vi "Tracking_End.vi"(6 "Last Frame Data":T3 {"Frame Data"."Image Type" items=["Grayscale (U8)", "Grayscale (I16)", "Grayscale (SGL)", "Complex (CSG)", "RGB (U32)", "HSL (U32)", "RGB (U64)", "Grayscale (U16)"]}, 7 "?":T1, 8 "error in":errorcluster, 9 "Settings":T5={"Harware Configuration"={"Camera"="cam1", "Frames Per Second"=15, "Simulate Recording"=FALSE, "Simulated Recording Sample"=path "", "Timestamp Method"=enum."Camera Timestamp"}, "Base Recording Path"=path "", "Type Of Recording"="", "Recording Codec"="", "TrackingSettings"={"Max Radius"=0, "Threshold"=255.0, "ROI"={"Left"=1, "Top"=1, "Right"=2, "Bottom"=0, "Rotation"=0.0}}, "Calibration"={"Pixel Width (X)"=1.0, "Pixel Height (Y)"=1.0}, "Broadcast Length"=0} {"Broadcast Length" min=0; "TrackingSettings"."ROI"."Rotation" format="%.2f"; "TrackingSettings"."ROI"."Left" scale=0.0..1024.0; "TrackingSettings"."ROI"."Right" scale=0.0..1024.0; "TrackingSettings"."Threshold" scale=0.0..255.0}, 10 "Output Data Queue":refnum<queue>, 11 "Input Data Queue":refnum<queue>) -> (0 "error out":errorcluster, 2 "Output Data Queue":refnum<queue>, 3 "Input Data Queue 2":refnum<queue>, 4 "Last Frame Data Out":T3 {"Frame Data"."Image Type" items=["Grayscale (U8)", "Grayscale (I16)", "Grayscale (SGL)", "Complex (CSG)", "RGB (U32)", "HSL (U32)", "RGB (U64)", "Grayscale (U16)"]}, 5 "?":T1)   [LabVIEW 2017, in "ImageAcquisitionLibrary.lvlib"]
uses:
  ImageAcquisitionLibrary.lvlib
  Acquisition/AcquireData.ctl
  Settings/Settings.ctl
  <vilib>/userdefined/High Color/IMAQdx.ctl
  TrackingSettings.ctl
  Settings/Calibration.ctl
  TrackingImages.ctl
  <vilib>/vision/Image Controls.llb/IMAQ Image.ctl
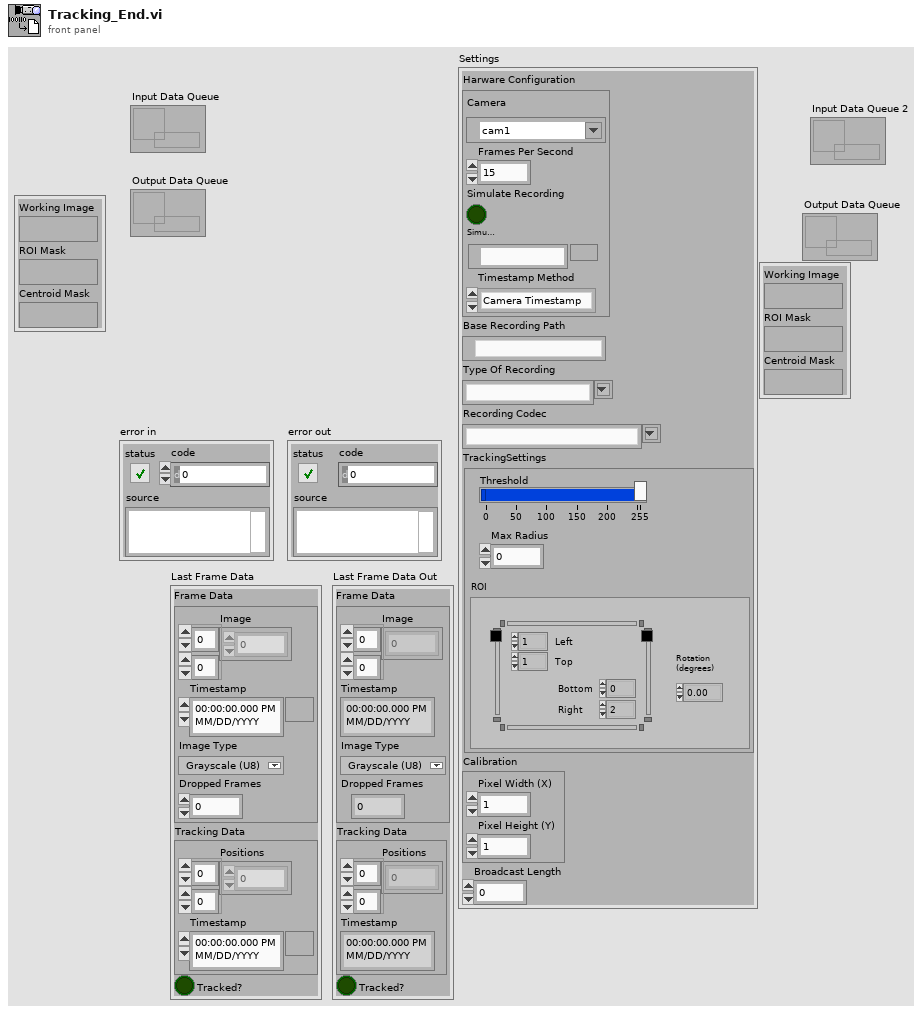
[diagram p1: front panel]
types:
  T1 = typedef "ImageAcquisitionLibrary.lvlib/TrackingImages.ctl" = cluster{"Working Image":T2, "ROI Mask":T2, "Centroid Mask":T2}
  T2 = typedef "IMAQ Image.ctl" = refnum<image>
  T3 = typedef "ImageAcquisitionLibrary.lvlib/AcquireData.ctl" = cluster{"Frame Data":cluster{"Image":u32[][], "Timestamp":timestamp, "Image Type":T4, "Dropped Frames":u32}, "Tracking Data":cluster{"Positions":dbl[][], "Timestamp":timestamp}, "Tracked?":bool}
  T4 = typedef "Image Type" = u32
  T5 = typedef "ImageAcquisitionLibrary.lvlib/Settings.ctl" = cluster{"Harware Configuration":cluster{"Camera":T6, "Frames Per Second":u32, "Simulate Recording":bool, "Simulated Recording Sample":path, "Timestamp Method":enum16{"System Timestamp", "Camera Timestamp", "IMAQdx Timestamp"}}, "Base Recording Path":path, "Type Of Recording":string, "Recording Codec":string, "TrackingSettings":T7, "Calibration":T9, "Broadcast Length":i32}
  T6 = typedef "IMAQdx.ctl" = refnum<k21>
  T7 = typedef "ImageAcquisitionLibrary.lvlib/TrackingSettings.ctl" = cluster{"Max Radius":i32, "Threshold":sgl, "ROI":T8}
  T8 = typedef "IMAQ Rectangle" = cluster{"Left":i32, "Top":i32, "Right":i32, "Bottom":i32, "Rotation":dbl}
  T9 = typedef "ImageAcquisitionLibrary.lvlib/Calibration.ctl" = cluster{"Pixel Width (X)":dbl, "Pixel Height (Y)":dbl}
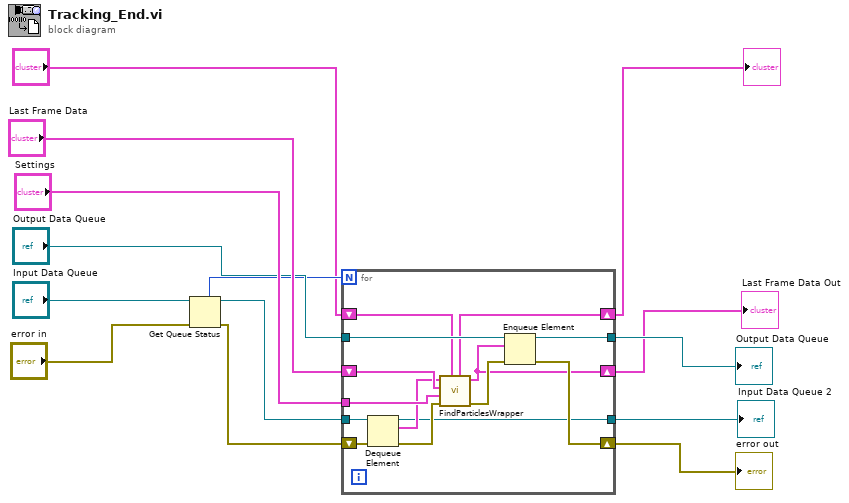
[diagram p0: block diagram]
diagram:
  n1 = Get Queue Status(queue="Input Data Queue", error in (no error)="error in") -> (queue out=w8:refnum<queue>, error out=w10:errorcluster, # elements in queue=w11:i32)  [unwired: 1 in, 5 out]
  n2 = for {
    N: w11 -> [_]
    shift-right: [w25] -> w6
    shift-left: w10 -> [w23]
    tunnel: "Settings" -> [w28]
    tunnel: w8 -> [w21]
    shift-right: [w17] -> w5
    shift-left: "Last Frame Data" -> [w27]
    tunnel: [w24] -> w9
    tunnel: [w19] -> w7
    tunnel: "Output Data Queue" -> [w18]
    shift-right: [w15] -> w1
    shift-left: "?" -> [w16]
    n3 = Dequeue Element(queue=w21, error in (no error)=w23) -> (queue out=w19:refnum<queue>, element=w20:T3, error out=w22:errorcluster)  [unwired: 1 in, 1 out]
    n4 = call "FindParticlesWrapper.vi"(7:w16, "error in"=w22, "Settings"=w28, "Data Old"=w27, "Data"=w20) -> ("error out"=w26:errorcluster, "Data Out"=w17:T3, 5:w15:T1)  [unwired: 4 in]
    n5 = Enqueue Element(queue=w18, element=w17, error in (no error)=w26) -> (queue out=w24:refnum<queue>, error out=w25:errorcluster)  [unwired: 1 in, 1 out]
  }
  "Last Frame Data Out" <- w5
  "error out" <- w6
  "Output Data Queue" <- w9
  "Input Data Queue 2" <- w7
  "?" <- w1
